vi "SystemCore Functions.vi"() -> ()   [LabVIEW 2026]
uses:
  vi.lib/MRC/MrcLib/MrcLib.lvlib
panel:
  out "Team Number":string
  out "input voltage (V)":dbl
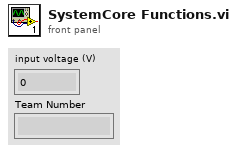
[diagram p1: front panel]
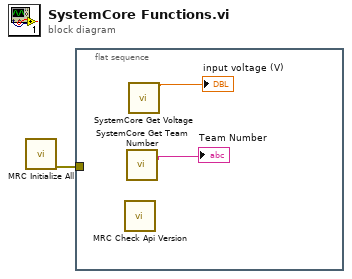
[diagram p0: block diagram]
diagram:
  n1 = call "MRC Initialize All.vi"() -> ("error out"=w1:errorcluster)  [unwired: 11 in]
  n2 = flat-sequence {
    tunnel: w1 -> [_]
    frame #0 {
      n3 = call "MRC Check Api Version.vi"() -> ()  [unwired: 10 in, 2 out]
      n4 = call "SystemCore Get Team Number.vi"() -> ("Team Number"=→"Team Number":string)  [unwired: 14 in, 1 out]
      n5 = call "SystemCore Get Voltage.vi"() -> ("input voltage (V)"=→"input voltage (V)":dbl)  [unwired: 14 in, 1 out]
    }
  }
